vi "State Formatting.vi"(11 "String 2":string) -> (3 "String":string)   [LabVIEW 2024]
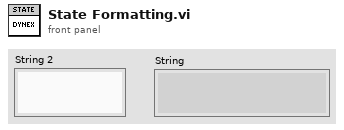
[diagram p1: front panel]
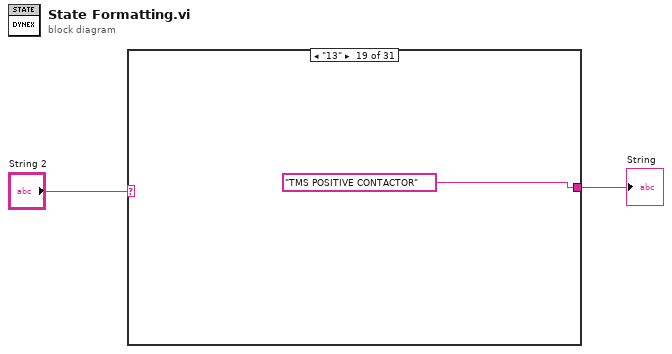
[diagram p0: block diagram]
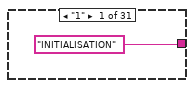
[diagram p2: hidden frame]
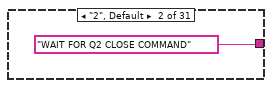
[diagram p3: hidden frame]
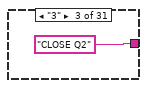
[diagram p4: hidden frame]
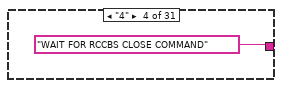
[diagram p5: hidden frame]
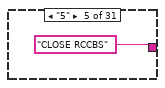
[diagram p6: hidden frame]
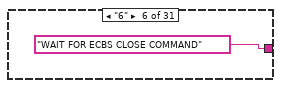
[diagram p7: hidden frame]
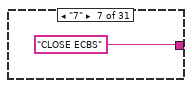
[diagram p8: hidden frame]
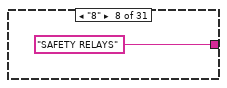
[diagram p9: hidden frame]
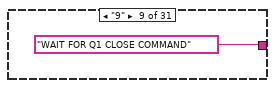
[diagram p10: hidden frame]
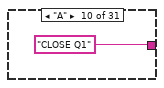
[diagram p11: hidden frame]
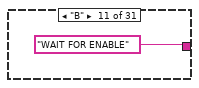
[diagram p12: hidden frame]
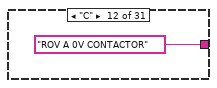
[diagram p13: hidden frame]
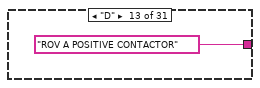
[diagram p14: hidden frame]
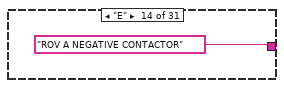
[diagram p15: hidden frame]
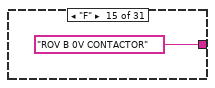
[diagram p16: hidden frame]
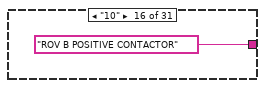
[diagram p17: hidden frame]
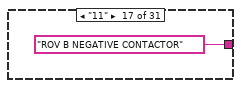
[diagram p18: hidden frame]
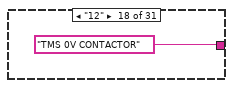
[diagram p19: hidden frame]
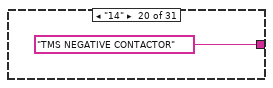
[diagram p20: hidden frame]
diagram:
  n1 = case shown="\"13\"" "String 2" {
    tunnel: ["INITIALISATION" ("String") "WAIT FOR Q2 CLOSE COMMAND" ("String") "CLOSE Q2" ("String") "WAIT FOR RCCBS CLOSE COMMAND" ("String") "CLOSE RCCBS" ("String") "WAIT FOR ECBS CLOSE COMMAND" ("String") "CLOSE ECBS" ("String") "SAFETY RELAYS" ("String") "WAIT FOR Q1 CLOSE COMMAND" ("String") "CLOSE Q1" ("String") "WAIT FOR ENABLE" ("String") "ROV A 0V CONTACTOR" ("String") "ROV A POSITIVE CONTACTOR" ("String") "ROV A NEGATIVE CONTACTOR" ("String") "ROV B 0V CONTACTOR" ("String") "ROV B POSITIVE CONTACTOR" ("String") "ROV B NEGATIVE CONTACTOR" ("String") "TMS 0V CONTACTOR" ("String") "TMS POSITIVE CONTACTOR" ("String") "TMS NEGATIVE CONTACTOR" ("String") "WAIT FOR START" ("String") "CLOSE K2" ("String") "CLOSE K1" ("String") "OPEN K2" ("String") "NORMAL OPERATION" ("String") "CONTROLLED SHUTDOWN" ("String") "EMERGENCY SHUTDOWN" ("String") "FAULT" ("String") "ROV A TRIP" ("String") "ROV B TRIP" ("String") "TMS TRIP" ("String")] -> w1
    frame "1" {
    }
    frame "2", Default {
    }
    frame "3" {
    }
    frame "4" {
    }
    frame "5" {
    }
    frame "6" {
    }
    frame "7" {
    }
    frame "8" {
    }
    frame "9" {
    }
    frame "A" {
    }
    frame "B" {
    }
    frame "C" {
    }
    frame "D" {
    }
    frame "E" {
    }
    frame "F" {
    }
    frame "10" {
    }
    frame "11" {
    }
    frame "12" {
    }
    frame "13" {
    }
    frame "14" {
    }
    frame "15" {
    }
    frame "16" {
    }
    frame "17" {
    }
    frame "18" {
    }
    frame "19" {
    }
    frame "1A" {
    }
    frame "1B" {
    }
    frame "1C" {
    }
    frame "1D" {
    }
    frame "1E" {
    }
    frame "1F" {
    }
  }
  "String" <- w1
